vi "GDSII Playground.vi"() -> ()   [LabVIEW 2019]
uses:
  ParseGDSII/ParseGDSII.lvclass
  Elements/Geometric.lvclass
  Fast Tree/Fast Tree.lvclass
panel:
  out "Visualized Tree":string
  out "Array 2":T1(array[cluster])
  out "Parse Structs":u32
  out "Find References":u32
  out "Tree Creation":u32
  out "Init Time":u32
  out "x-y":u32
  out "error out":errorcluster
  out "XY Graph":cluster{"X":i32[], "Y":i32[]}[](graph)
  in  "error in (no error)":errorcluster
  in  "Path":path=path "C:/Users/Albro/Documents/GitHub/AFM-Lithography/lvsrc/Classes/Parse/GDSII/test files/example.gds"
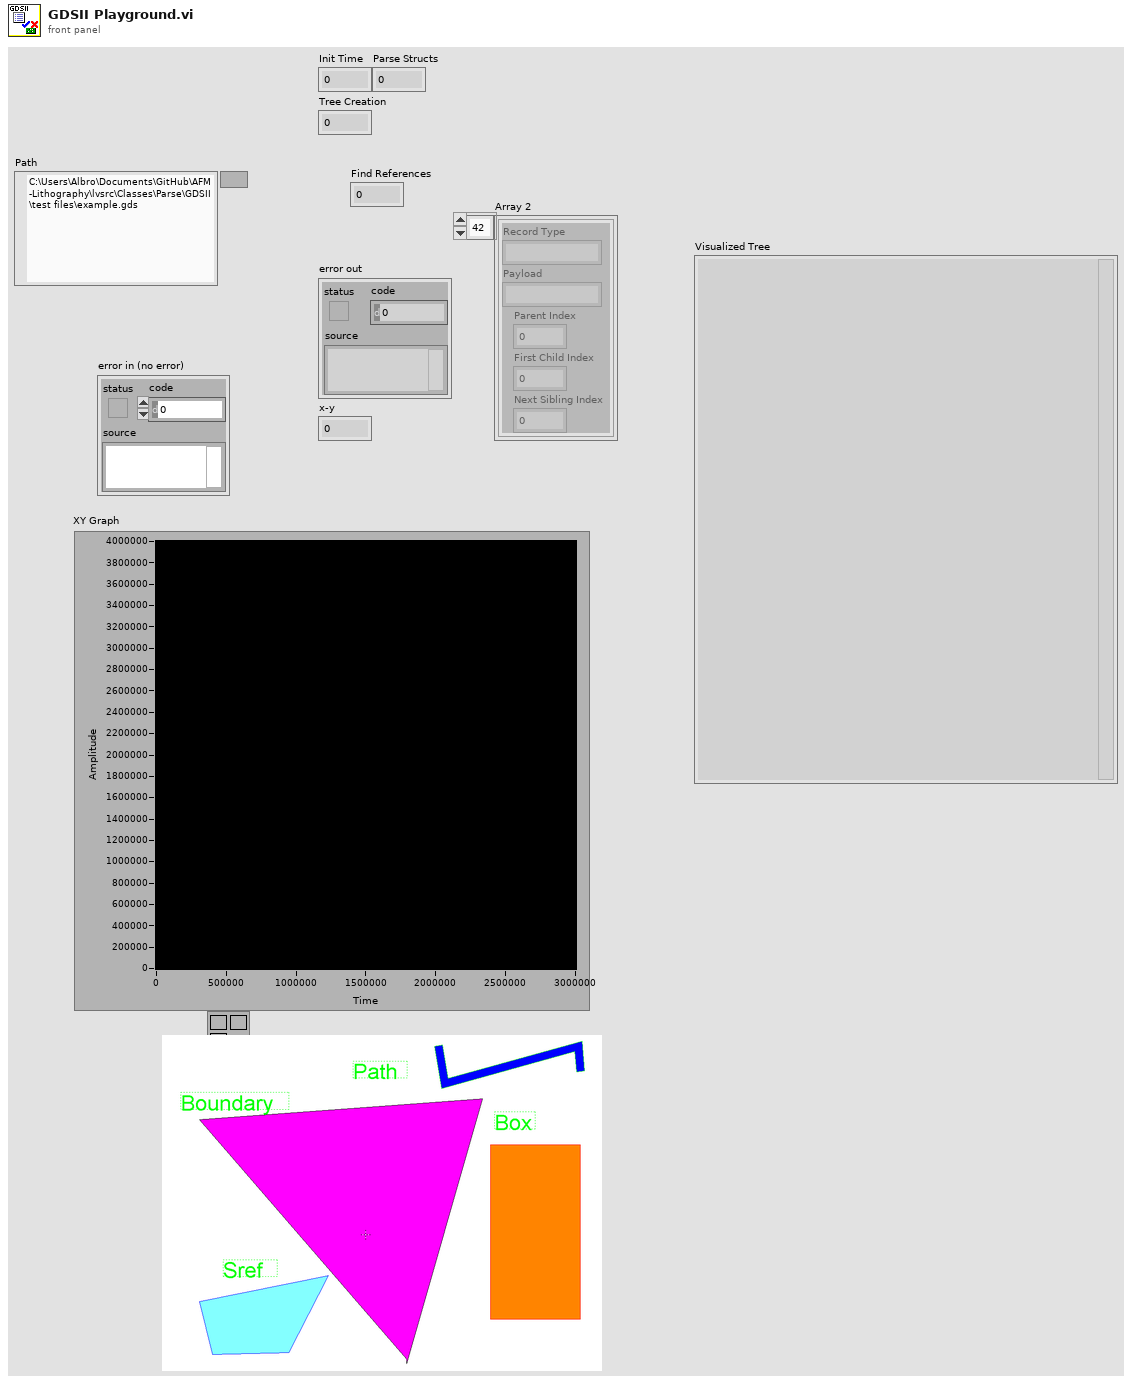
[diagram p1: front panel]
types:
  T1 = cluster{"Record Type":string, "Payload":string, "Parent Index":i32, "First Child Index":i32, "Next Sibling Index":i32}[]
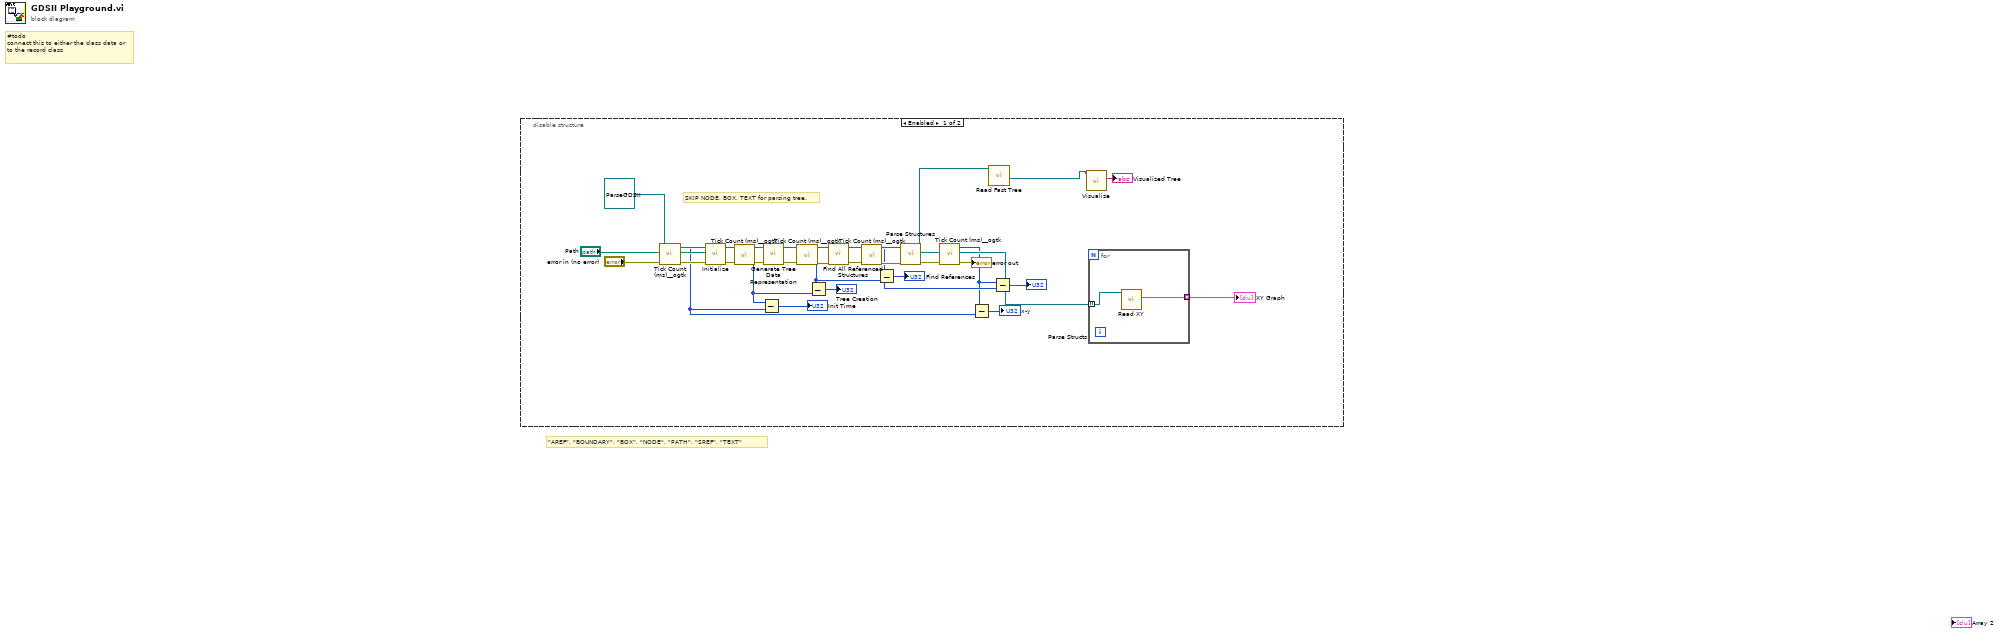
[diagram p0: block diagram]
diagram:
  # "\"AREF\", \"BOUNDARY\", \"BOX\", \"NODE\", \"PATH\", \"SREF\", \"TEXT\""
  # "#todo\nconnect this to either the class data or to the record class"
  n1 = disable-structure shown="Enabled" {
    frame Enabled {
      # "SKIP NODE, BOX, TEXT for parsing tree."
      n2 = call <userlib>:"Tick Count (ms)__ogtk.vi"("error in (no error)"="error in (no error)") -> ("error out"=w21:errorcluster, "millisecond timer value"=w17:u32)  [unwired: 9 in]
      n3 = call "Initialize.vi"("error in (no error)"=w21, "Path"="Path", "ParseGDSII in"=refnum<class "ParseGDSII.lvclass"> refnum) -> ("error out"=w19:errorcluster, "ParseGDSII out"=w28:refnum<class "ParseGDSII.lvclass">)  [unwired: 7 in]
      n4 = call <userlib>:"Tick Count (ms)__ogtk.vi"("error in (no error)"=w19) -> ("error out"=w18:errorcluster, "millisecond timer value"=w13:u32)  [unwired: 9 in]
      n5 = Subtract(x=w13, y=w17) -> (x-y=→"Init Time":u32)
      n6 = call "Generate Tree Data Representation.vi"("error in (no error)"=w18, "ParseGDSII in"=w28) -> ("error out"=w15:errorcluster, "ParseGDSII out"=w27:refnum<class "ParseGDSII.lvclass">)  [unwired: 8 in]
      n7 = call <userlib>:"Tick Count (ms)__ogtk.vi"("error in (no error)"=w15) -> ("error out"=w14:errorcluster, "millisecond timer value"=w8:u32)  [unwired: 9 in]
      n8 = Subtract(x=w8, y=w13) -> (x-y=→"Tree Creation":u32)
      n9 = call "Find All Referenced Structures.vi"("error in"=w14, "ParseGDSII in"=w27) -> ("error out"=w10:errorcluster, "ParseGDSII out"=w30:refnum<class "ParseGDSII.lvclass">)  [unwired: 8 in]
      n10 = call <userlib>:"Tick Count (ms)__ogtk.vi"("error in (no error)"=w10) -> ("error out"=w9:errorcluster, "millisecond timer value"=w7:u32)  [unwired: 9 in]
      n11 = Subtract(x=w7, y=w8) -> (x-y=→"Find References":u32)
      n12 = call "Parse Structures.vi"("error in"=w9, "ParseGDSII in"=w30) -> ("error out"=w24:errorcluster, "Geometric"=w29:refnum<class "Geometric.lvclass">[], "ParseGDSII out"=w3:refnum<class "ParseGDSII.lvclass">)  [unwired: 7 in]
      n13 = call <userlib>:"Tick Count (ms)__ogtk.vi"("error in (no error)"=w24) -> ("error out"=→"error out":errorcluster, "millisecond timer value"=w6:u32)  [unwired: 9 in]
      n14 = Subtract(x=w6, y=w17) -> (x-y=→"x-y":u32)
      n15 = call "Read Fast Tree.vi"("ParseGDSII in"=w3) -> ("Fast Tree.lvclass"=w1:refnum<class "Fast Tree.lvclass">)  [unwired: 7 in, 3 out]
      n16 = Subtract(x=w6, y=w7) -> (x-y=→"Parse Structs":u32)
      n17 = call "Visualize.vi"("Fast Tree in"=w1) -> ("Visualized Tree"=→"Visualized Tree":string)  [unwired: 8 in, 2 out]
      n18 = for {
        tunnel: w29 -> [w32] mode=indexing
        tunnel: [w31] -> w4 mode=indexing
        n19 = call-dynamic "Read XY.vi"("Element in"=w32) -> ("XY"=w31:cluster{"X":i32[], "Y":i32[]})  [unwired: 8 in, 2 out]
      }
      "XY Graph" <- w4
    }
    frame Disabled {
    }
  }
